vi "Signal Detect.vi"() -> ()   [LabVIEW 2016]
uses:
  Source/GE 5565PIORC/GE 5565PIORC.lvclass/GE 5565PIORC.ctl
  Source/GE 5565PIORC/VIs/Registers/Local Configuration.LAS1RR.Address Range.Get.vi
  Source/GE 5565PIORC/VIs/Binary Operations/Get Bits.vi
  Source/GE 5565PIORC/VIs/Binary Operations/Get Bits U32.vi
  Source/GE 5565PIORC/VIs/Registers/RFM Control and Status.Get Register Offset.vi
  Source/GE 5565PIORC/VIs/Registers/Local Configuration.Get Register Offset.vi
  Source/GE 5565PIORC/GE 5565PIORC.lvclass
panel:
  out "RX Signal Detected?":bool
  in  "stop":bool
  in  "VISA resource name":refnum<visa-resource-name>
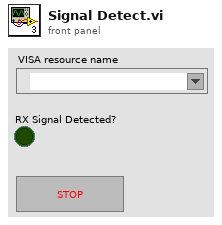
[diagram p1: front panel]
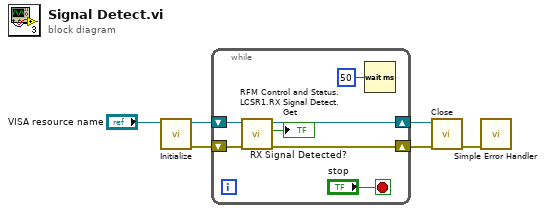
[diagram p0: block diagram]
diagram:
  n1 = call "Initialize.vi"("VISA resource name"="VISA resource name") -> ("error out"=w3:errorcluster, "GE 5565PIORC"=w4:refnum<class "GE 5565PIORC.lvclass">)  [unwired: 9 in]
  n2 = while {
    shift-right: [w11] -> w2
    shift-left: w4 -> [w13]
    shift-right: [w10] -> w1
    shift-left: w3 -> [w12]
    stop <- "stop" stop-if-true
    n3 = call "RFM Control and Status.LCSR1.RX Signal Detect.Get.vi"("error in (no error)"=w12, "GE 5565PIORC"=w13) -> ("error out"=w10:errorcluster, "RX Signal Detected?"=→"RX Signal Detected?":bool, "GE 5565PIORC out"=w11:refnum<class "GE 5565PIORC.lvclass">)  [unwired: 7 in]
    n4 = Wait (ms)(milliseconds to wait=u32 50) -> ()  [unwired: 1 out]
  }
  n5 = call "Close.vi"("error in (no error)"=w1, "GE 5565PIORC in"=w2) -> ("error out"=w5:errorcluster)  [unwired: 8 in, 1 out]
  n6 = call <vilib>:"Simple Error Handler.vi"("error in (no error)"=w5) -> ()  [unwired: 4 in, 5 out]
